vi "SVT UFF58 Write.vi"   [LabVIEW 2017, in "SoundVib_UFF58.lvlib"]
doc: "Writes data to the UFF58 (universal file format) file specified by the <B>file refnum</B> input. This VI also writes the fields in records 1, 2, and 3, <B>ID lines (1-3)</B>. You can write a single time domain waveform, multiple time domain waveforms, a single real frequency spectrum, multiple real frequency spectra, a single complex frequency spectrum, multiple complex frequency spectra, or generic data to a UFF file. If a frequency spectrum is in decibels, this VI converts the spectrum to linear before writing to the UFF58 file. The default instance, SVT UFF58 Write Time Waveform (1 Ch), writes a single time domain waveform to the file specified by the <B>file refnum</B> input. Wire data to the <B>file refnum</B> input to determine the polymorphic instance to use or manually select the instance."
uses:
  <vilib>/addons/Sound and Vibration/svt_UFF58/SoundVib_UFF58.lvlib
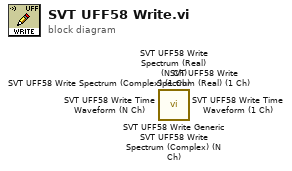
[diagram p0: block diagram]
diagram:
  n1 = call <vilib>:"SVT UFF58 Write Generic.vi"() -> ()  [unwired: 13 in, 3 out]
  n2 = call <vilib>:"SVT UFF58 Write Spectrum (Real) (1 Ch).vi"() -> ()  [unwired: 13 in, 3 out]
  n3 = call <vilib>:"SVT UFF58 Write Time Waveform (N Ch).vi"() -> ()  [unwired: 13 in, 3 out]
  n4 = call <vilib>:"SVT UFF58 Write Time Waveform (1 Ch).vi"() -> ()  [unwired: 13 in, 3 out]
  n5 = call <vilib>:"SVT UFF58 Write Spectrum (Complex) (N Ch).vi"() -> ()  [unwired: 13 in, 3 out]
  n6 = call <vilib>:"SVT UFF58 Write Spectrum (Complex) (1 Ch).vi"() -> ()  [unwired: 13 in, 3 out]
  n7 = call <vilib>:"SVT UFF58 Write Spectrum (Real) (N Ch).vi"() -> ()  [unwired: 13 in, 3 out]
